vi "SCP Set Permissions Test.vi"() -> ()   [LabVIEW 2013]
uses:
  SCP File Transfer.lvclass
panel:
  out "Error?":bool
  out "error out":errorcluster
  in  "Remote path":string
  in  "Address":string
  in  "Username":string
  in  "Password":string
  # "Test 1: Set permissions on a file no error"
  # "Test 2: Set permissions with wrong file name - should get chmod error"
  # "Test 3: Use bad address - should get timeout"
  # "Test 4: use bad admin or password"
  # "Test 5: Turn off ssh in max, should get prompt to enable ssh"
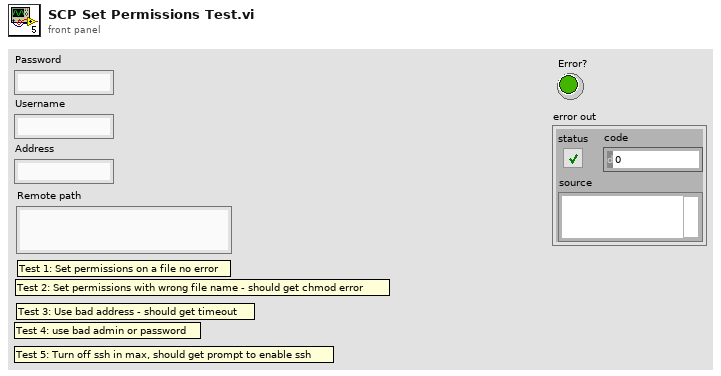
[diagram p1: front panel]
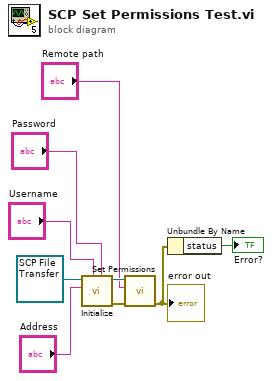
[diagram p0: block diagram]
diagram:
  n1 = call-dynamic "Initialize.vi"("Password"="Password", "Username"="Username", "Address"="Address", "SCP File Transfer in"=refnum<class "SCP File Transfer.lvclass"> refnum) -> ("error out"=w7:errorcluster, "SCP File Transfer out"=w8:refnum<class "SCP File Transfer.lvclass">)  [unwired: 6 in]
  n2 = call "Set Permissions.vi"("error in (no error)"=w7, "Remote path"="Remote path", "SCP File Transfer in"=w8) -> ("error out"=w2:errorcluster)  [unwired: 7 in, 1 out]
  "error out" <- w2
  n3 = Unbundle By Name(w2) -> ("status"=→"Error?":bool)
